vi "run_experiment_sCMOS_DAC_DEBUG.vi"() -> ()   [LabVIEW 2015]
uses:
  <vilib>/DAQmx/read.llb/DAQmx Read (Analog 1D Wfm NChan NSamp).vi
  <vilib>/DAQmx/write.llb/DAQmx Write (Digital Bool 1Line 1Point).vi
  <vilib>/DAQmx/create/channels.llb/DAQmx Create Channel (DO-Digital Output).vi
  <vilib>/DAQmx/miscellaneous.llb/DAQmx Fill In Error Info.vi
  <vilib>/DAQmx/create/channels.llb/DAQmx Create Channel (AI-Voltage-Basic).vi
  <vilib>/DAQmx/configure/timing.llb/DAQmx Timing (Sample Clock).vi
panel:
  out "Display":T1(plugin-control)
  out "DAC Input":waveform(dbl)[](graph) caption="DAC Input Display"
  out "Frames Recorded":i32
  out "error out":errorcluster
  out "Current Stimulus Name":string
  out "Current Piezo Command":dynamicdata(graph)
  out "Acquiring Frames":bool
  out "Current Stim Frames":dbl
  out "Current Stim Duration":dbl
  out "Current Stimulus Save Path":path
  in  "Number Reps":dbl
  out "Experiment Path":path
  out "Timestamp":string
  out "Genotype":string
  out "Fly Name":string
  out "Experiment Name":string
  in  "Metadata Path":path
  out "Stimulus Files":path[](array[path])
  out "Num Stimuli":i32
  out "Protocol Name":string
  out "Protocol Rate":i32
  in  "Protocol Path":path
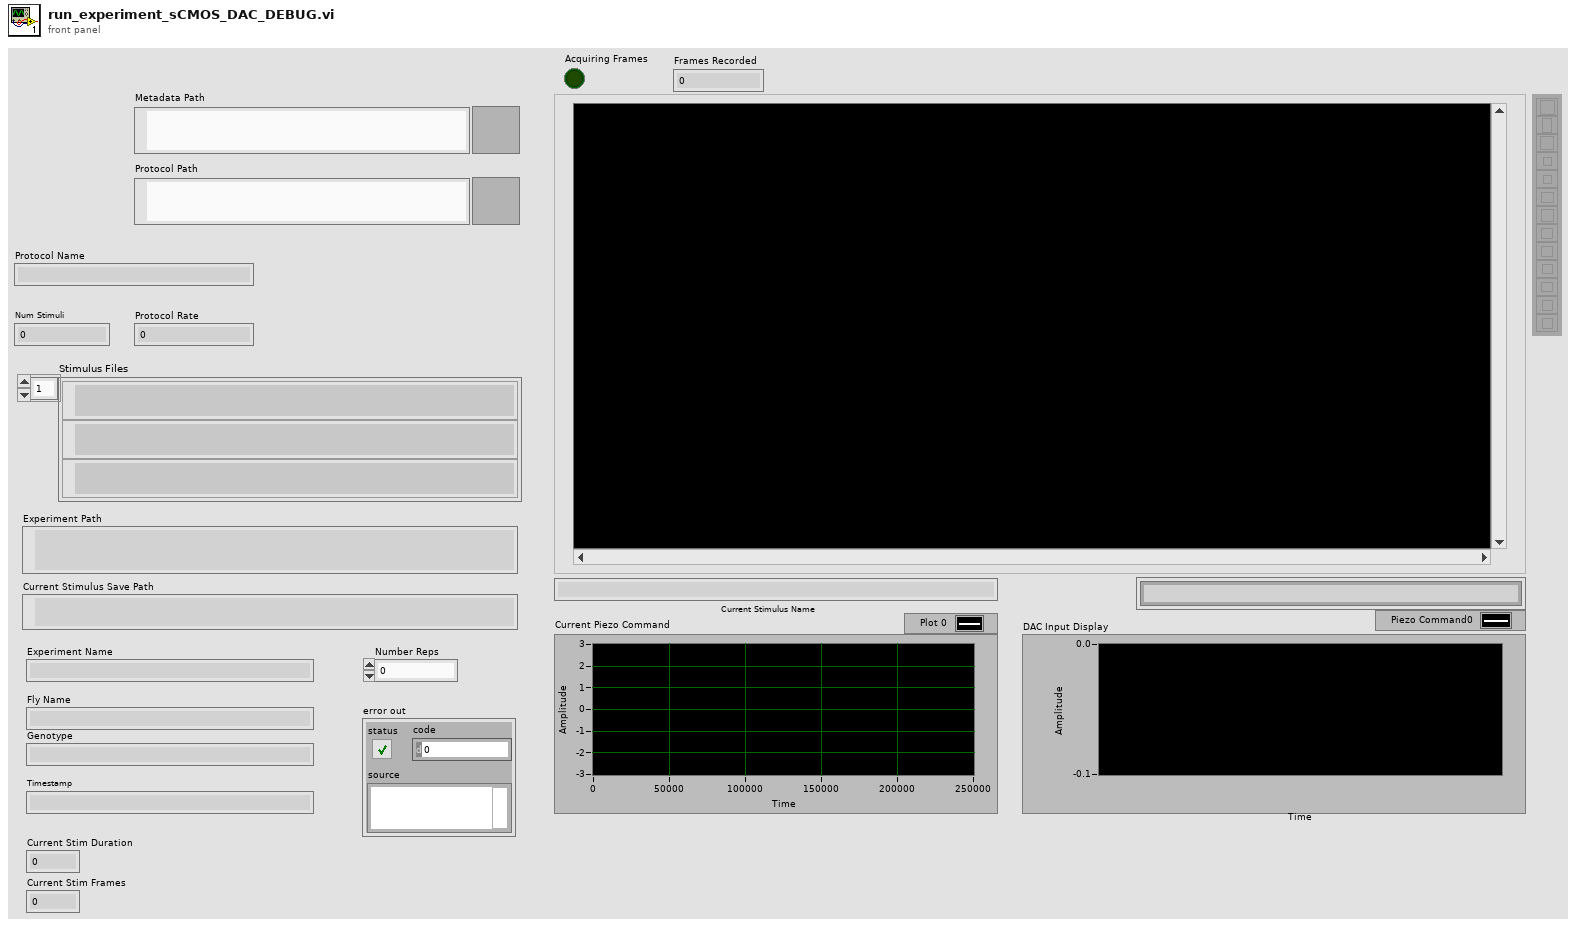
[diagram p1: front panel]
types:
  T1 = typedef "IMAQ Image.ctl" = refnum<image>
  T2 = cluster{"Value":i32, "Minimum":i32, "Maximum":i32, "Increment":i32}
  T3 = typedef "Image Type" = u32
  T4 = cluster{"height":u32, "width":u32, "datatype":u32}
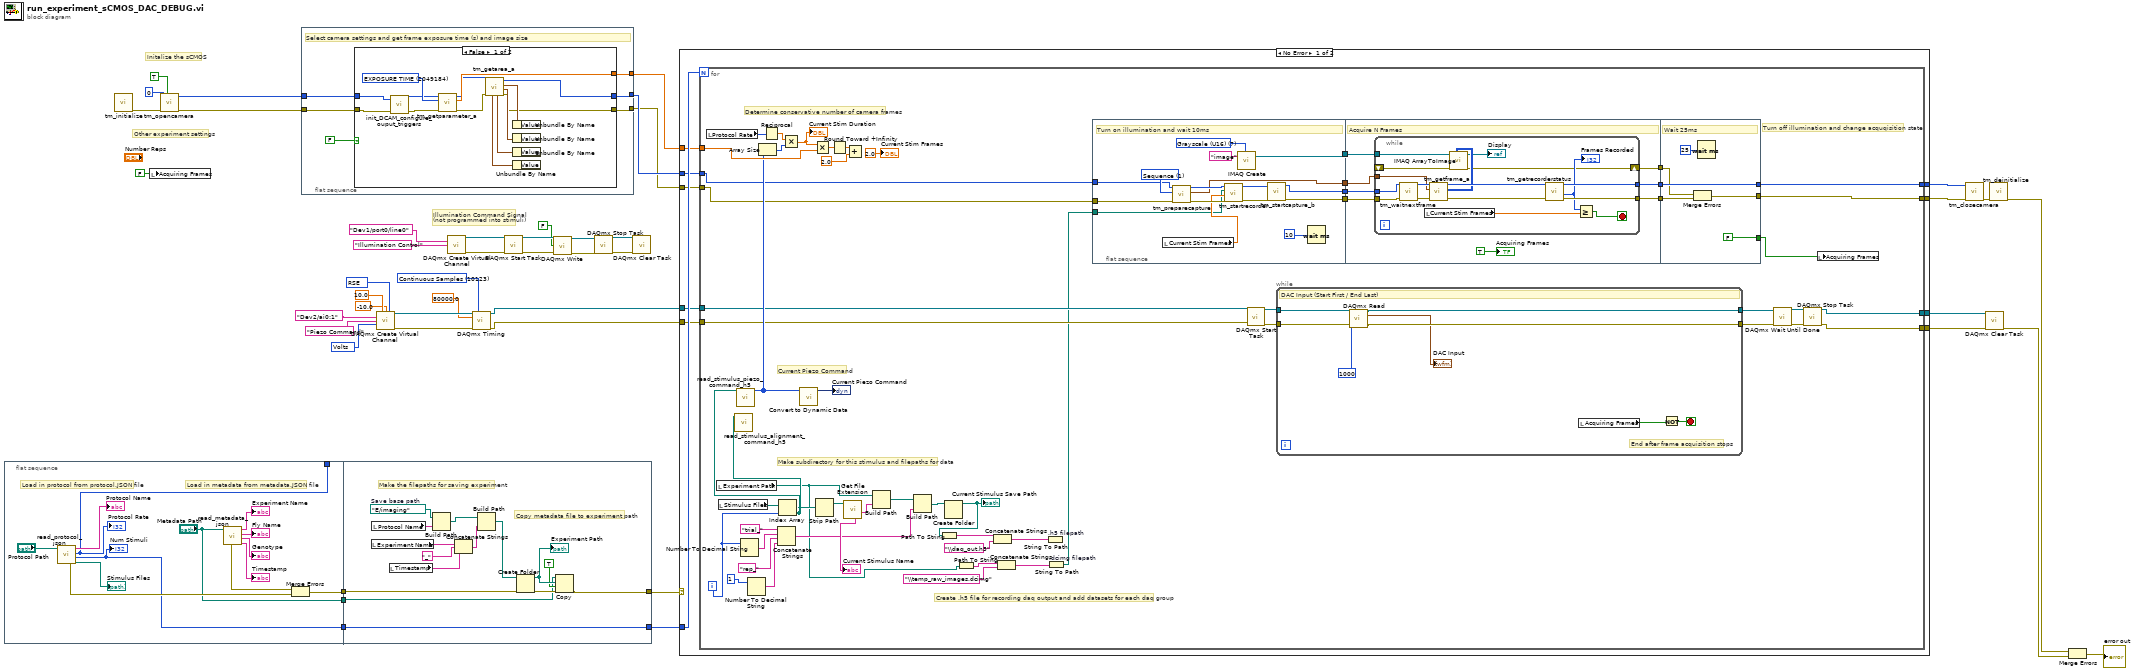
[diagram p0: block diagram]
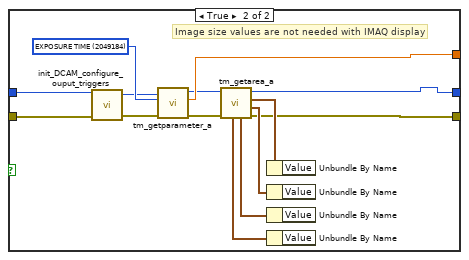
[diagram p3: hidden frame]
diagram:
  w8 = 10083 items=["default"=-1, "RSE"=10083, "NRSE"=10078, "Differential"=10106, "Pseudodifferential"=12529] ("input terminal configuration")
  w9 = 10123 items=["Finite Samples"=10178, "Continuous Samples"=10123] ("sample mode")
  w10 = 10348 items=["Volts"=10348, "From Custom Scale"=10065] ("units")
  # "Other experiment settings"
  # "Initalize the sCMOS"
  # "Illumination Command Signal \n(not programmed into stimuli)"
  n1 = flat-sequence {
    tunnel: [w48] -> _
    tunnel: [w49] -> w21
    tunnel: ["Metadata Path"] -> w20
    tunnel: [w46] -> w19
    tunnel: [w73] -> w39
    tunnel: w21 -> [w61]
    tunnel: w20 -> [w60]
    tunnel: w19 -> [w73]
    tunnel: [w59] -> w18
    frame #0 {
      # "Load in metadata from metadata.JSON file"
      # "Load in protocol from protocol.JSON file"
      n2 = call "read_protocol_json.vi"("Path"="Protocol Path") -> ("stims"=→"Stimulus Files":path[], "n_stims"=w46:i32, "rate"=w48:i32, "protocol name"=→"Protocol Name":string, "error out"=w51:errorcluster)  [unwired: 6 in]
      "Protocol Rate" <- w48
      "Num Stimuli" <- w46
      n3 = call "read_metadata_json.vi"("Path"="Metadata Path") -> ("exp_time"=→"Timestamp":string, "genotype"=→"Genotype":string, "fly_name"=→"Fly Name":string, "exp_ name"=→"Experiment Name":string, "error out"=w50:errorcluster)  [unwired: 6 in]
      n4 = Merge Errors(w50, w51) -> (w49:errorcluster)
    }
    frame #1 {
      w68 = path "E:/imaging"  # Save base path
      # "Copy metadata file to experiment path"
      # "Make the filepaths for saving experiment"
      n5 = local read "Experiment Name"() -> (w65:string)
      n6 = local read "Protocol Name"() -> (w67:string)
      n7 = local read "Timestamp"() -> (w63:string)
      n8 = Build Path(base path=w68, name or relative path=w67) -> (appended path=w66:path)
      n9 = Concatenate Strings(w65, "_", w63) -> (w62:string)
      n10 = Build Path(base path=w66, name or relative path=w62) -> (appended path=w69:path)
      n11 = Create Folder(path (use dialog)=w69, error in=w61) -> (created path=w72:path, error out=w71:errorcluster)  [unwired: 1 in, 1 out]
      "Experiment Path" <- w72
      n12 = Copy(8:w71, 9:TRUE ("overwrite (F)"), 10:w72, 11:w60) -> (0:w59:errorcluster)  [unwired: 1 in, 2 out]
    }
  }
  n13 = call <userlib>:"tm_initialize.vi"() -> ("error out"=w42:errorcluster)  [unwired: 8 in, 3 out]
  n14 = local write "Acquiring Frames"(FALSE ("Acquiring Frames")) -> ()
  n15 = call <userlib>:"tm_opencamera.vi"("Force Open"=TRUE, "error in (no error)"=w42, "Camera Index"=0) -> ("error out"=w29:errorcluster, "Handle out"=w30:u32)  [unwired: 6 in, 1 out]
  n16 = flat-sequence {
    tunnel: [w76] -> w32
    tunnel: [w75] -> w24
    tunnel: [w79] -> w31
    tunnel: w30 -> [w78]
    tunnel: w29 -> [w77]
    frame #0 {
      # "Select camera settings and get frame exposure time (s) and image size"
      n17 = case shown="False" FALSE {
        tunnel: [w92 w106] -> w79
        tunnel: w78 -> [w80 w97]
        tunnel: w77 -> [w83 w96]
        tunnel: [w85 w95] -> w76
        tunnel: [w84 w94] -> w75
        frame False {
          w93 = u32 2049184 items=["SENSOR MODE"=4212128, "CCD MODE"=4212384, "READOUT MODE"=4211872, "ACTIVE VIEW INDEX"=4343136, "BITS PER CHANNEL"=4342976, "IMAGE PIXEL TYPE"=4343296, "BINNING"=4215968, "EXPOSURE TIME"=2049184, "CONTRAST GAIN"=3163312, "CONTRAST OFFSET"=3163328, "LIGHT MODE"=2114720, "SENSITIVITY"=2114992, "PHOTON IMAGING MODE"=2115200, "HIGH DYNAMIC RANGE MODE"=3163360, "WHITE BALANCE"=3163568, "TEMPERATURE"=2115232, "TEMPERATURE TARGET"=2115264, "SENSOR COOLER FAN"=2115296, "LINEBUNDLE HEIGHT"=4212192, "MECHANICAL SHUTTER"=2115488, "BACK FOCUS POSITION"=8422304, "TRIGGER CONNECTOR"=1066432, "TRIGGER SOURCE"=1066144, "OUTPUT TRIGGER SOURCE"=1852576, "TRIGGER GLOBAL EXPOSURE"=2049680, "FIRST TRIGGER BEHAVIOR"=2049696, "CHANNEL SYNC"=1852352, "READOUT DIRECTION"=4211904, "PRE HSYNC COUNT"=1852704] ("Parameter")
          n18 = call "init_DCAM_configure_ouput_triggers.vi"("error in (no error)"=w83, "Handle in"=w80) -> ("error out"=w82:errorcluster, "Handle out"=w81:u32)  [unwired: 2 in]
          n19 = call <userlib>:"tm_getparameter_a.vi"("error in (no error)"=w82, "Parameter"=w93, "Handle in"=w81) -> ("error out"=w87:errorcluster, "Value out"=w92:dbl, "Handle out"=w86:u32)  [unwired: 6 in]
          n20 = call <userlib>:"tm_getarea_a.vi"("error in (no error)"=w87, "Handle in"=w86) -> ("error out"=w84:errorcluster, "V Offset"=w90:T2, "H Offset"=w91:T2, "Handle out"=w85:u32, "H Width"=w89:T2, "V Width"=w88:T2)  [unwired: 4 in]
          n21 = Unbundle By Name(w91) -> ()  [unwired: 1 out]
          n22 = Unbundle By Name(w90) -> ()  [unwired: 1 out]
          n23 = Unbundle By Name(w89) -> ()  [unwired: 1 out]
          n24 = Unbundle By Name(w88) -> ()  [unwired: 1 out]
        }
        frame True {
          w107 = u32 2049184 items=["SENSOR MODE"=4212128, "CCD MODE"=4212384, "READOUT MODE"=4211872, "ACTIVE VIEW INDEX"=4343136, "BITS PER CHANNEL"=4342976, "IMAGE PIXEL TYPE"=4343296, "BINNING"=4215968, "EXPOSURE TIME"=2049184, "CONTRAST GAIN"=3163312, "CONTRAST OFFSET"=3163328, "LIGHT MODE"=2114720, "SENSITIVITY"=2114992, "PHOTON IMAGING MODE"=2115200, "HIGH DYNAMIC RANGE MODE"=3163360, "WHITE BALANCE"=3163568, "TEMPERATURE"=2115232, "TEMPERATURE TARGET"=2115264, "SENSOR COOLER FAN"=2115296, "LINEBUNDLE HEIGHT"=4212192, "MECHANICAL SHUTTER"=2115488, "BACK FOCUS POSITION"=8422304, "TRIGGER CONNECTOR"=1066432, "TRIGGER SOURCE"=1066144, "OUTPUT TRIGGER SOURCE"=1852576, "TRIGGER GLOBAL EXPOSURE"=2049680, "FIRST TRIGGER BEHAVIOR"=2049696, "CHANNEL SYNC"=1852352, "READOUT DIRECTION"=4211904, "PRE HSYNC COUNT"=1852704] ("Parameter")
          # "Image size values are not needed with IMAQ display"
          n25 = call "init_DCAM_configure_ouput_triggers.vi"("error in (no error)"=w96, "Handle in"=w97) -> ("error out"=w105:errorcluster, "Handle out"=w104:u32)  [unwired: 2 in]
          n26 = call <userlib>:"tm_getparameter_a.vi"("error in (no error)"=w105, "Parameter"=w107, "Handle in"=w104) -> ("error out"=w102:errorcluster, "Value out"=w106:dbl, "Handle out"=w103:u32)  [unwired: 6 in]
          n27 = call <userlib>:"tm_getarea_a.vi"("error in (no error)"=w102, "Handle in"=w103) -> ("error out"=w94:errorcluster, "V Offset"=w100:T2, "H Offset"=w101:T2, "Handle out"=w95:u32, "H Width"=w99:T2, "V Width"=w98:T2)  [unwired: 4 in]
          n28 = Unbundle By Name(w101) -> ()  [unwired: 1 out]
          n29 = Unbundle By Name(w100) -> ()  [unwired: 1 out]
          n30 = Unbundle By Name(w99) -> ()  [unwired: 1 out]
          n31 = Unbundle By Name(w98) -> ()  [unwired: 1 out]
        }
      }
    }
  }
  n32 = call-poly <vilib>:"DAQmx Create Virtual Channel.vi"("maximum value"=10.0, "minimum value"=-10.0, "input terminal configuration"=w8, "physical channels"=tag "Dev2/ai0:1" ("DAQmx Physical Channel"), "name to assign"="Piezo Command", "units"=w10) -> ("task out"=w16:refnum<k21>, "error out"=w17:errorcluster)  [unwired: 8 in]
  n33 = call-poly <vilib>:"DAQmx Create Virtual Channel.vi"("lines"=tag "Dev1/port0/line0" ("DAQmx Physical Channel"), "name to assign"="Illumination Control") -> ("task out"=w36:refnum<k21>, "error out"=w38:errorcluster)  [unwired: 12 in]
  n34 = call-poly <vilib>:"DAQmx Timing.vi"("task/channels in"=w16, "sample mode"=w9, "rate"=80000.0, "error in"=w17) -> ("task out"=w7:refnum<k21>, "error out"=w6:errorcluster)  [unwired: 10 in]
  n35 = call <vilib>:"DAQmx Start Task.vi"("task/channels in"=w36, "error in"=w38) -> ("task out"=w35:refnum<k21>, "error out"=w37:errorcluster)  [unwired: 12 in]
  n36 = call-poly <vilib>:"DAQmx Write.vi"("task/channels in"=w35, "data"=FALSE, "error in"=w37) -> ("task out"=w5:refnum<k21>, "error out"=w4:errorcluster)  [unwired: 10 in, 1 out]
  n37 = call <vilib>:"DAQmx Stop Task.vi"("task/channels in"=w5, "error in"=w4) -> ("task out"=w2:refnum<k21>, "error out"=w3:errorcluster)  [unwired: 12 in]
  n38 = call <vilib>:"DAQmx Clear Task.vi"("task in"=w2, "error in"=w3) -> ()  [unwired: 13 in, 1 out]
  n39 = case shown="No Error" w18 {
    tunnel: w39 -> [w117 _]
    tunnel: w31 -> [w116 _]
    tunnel: w32 -> [w115 w230]
    tunnel: w24 -> [w114 w229]
    tunnel: [w113 w229] -> w26
    tunnel: [w112 w230] -> w25
    tunnel: [w111 _] -> w23
    tunnel: [w110 _] -> w22
    tunnel: w7 -> [w109 _]
    tunnel: w6 -> [w108 _]
    frame No Error {
      n40 = for {
        N: w117 -> [_]
        tunnel: w116 -> [w161]
        tunnel: w115 -> [w131]
        tunnel: w114 -> [w130]
        tunnel: [w147] -> w113
        tunnel: [w146] -> w112
        tunnel: [w136] -> w111
        tunnel: [w135] -> w110
        tunnel: w109 -> [w134]
        tunnel: w108 -> [w133]
        i -> [w170]
        # "Create .h5 file for recording daq output and add datasets for each daq group"
        # "Current Piezo Command"
        # "Turn off illumination and change acquqisition state"
        # "Determine conservative number of camera frames"
        # "Make subdirectory for this stimulus and filepaths for data"
        n41 = local read "Protocol Rate"() -> (w165:i32)
        n42 = local read "Experiment Path"() -> (w122:path)
        n43 = local read "Stimulus Files"() -> (w171:path[])
        n44 = Number To Decimal String(number=w170) -> (decimal integer string=w173:string)  [unwired: 1 in]
        n45 = Number To Decimal String(number=i16 1 ("width (-)")) -> (decimal integer string=w168:string)  [unwired: 1 in]
        n46 = Reciprocal(x=w165) -> (1/x=w163:dbl)
        n47 = Concatenate Strings("trial_", w173, "rep_", w168) -> (w123:string)
        n48 = Index Array(array=w171, index=w170) -> (element=w166:path)
        n49 = call "read_stimulus_alignment_command_h5.vi"("Path"=w166) -> ()  [unwired: 9 in, 2 out]
        n50 = call "read_stimulus_piezo_command_h5.vi"("Path"=w166) -> ("stimulus"=w141:i32[])  [unwired: 9 in, 1 out]
        n51 = Array Size(array=w141) -> (size(s)=w164:i32)
        n52 = Multiply(x=w163, y=w164) -> (x*y=w162:dbl)
        "Current Stim Duration" <- w162
        n53 = call "Convert to Dynamic Data"("Array"=w141) -> ("Dynamic Data Type"=→"Current Piezo Command":dynamicdata)  [unwired: 3 in]
        n54 = Multiply(x=w162, y=w161) -> (x*y=w160:dbl)
        n55 = Strip Path(path=w166) -> (stripped path=w129:path)  [unwired: 1 out]
        n56 = Round Toward +Infinity(x=w160) -> (ceil(x): smallest int >= x=w159:dbl)
        n57 = call <vilib>:"Get File Extension.vi"("file"=w129) -> ("filename without extension"=w128:string, "unmodified file extension"=→"Current Stimulus Name":string)  [unwired: 6 in, 3 out]
        n58 = Add(x=w159, y=2.0) -> ()  [unwired: 1 out]
        n59 = Build Path(base path=w122, name or relative path=w128) -> (appended path=w125:path)
        n60 = Build Path(base path=w125, name or relative path=w123) -> (appended path=w124:path)
        n61 = Create Folder(path (use dialog)=w124) -> (created path=w126:path)  [unwired: 2 in, 2 out]
        "Current Stimulus Save Path" <- w126
        n62 = Path To String(path=w126) -> (string=w156:string)
        n63 = Path To String(path=w122) -> (string=w121:string)
        n64 = Concatenate Strings(w156, "\\daq_out.h5" ("string")) -> (w157:string)
        n65 = Concatenate Strings(w121, "\\temp_raw_images.dcimg" ("string")) -> (w119:string)
        n66 = String To Path ".h5 filepath"(string=w157) -> ()  [unwired: 1 out]
        n67 = String To Path ".dcimg filepath"(string=w119) -> (path=w118:path)
        n68 = flat-sequence {
          tunnel: [w181] -> w152
          tunnel: [w179] -> w151
          tunnel: [w180] -> w150
          tunnel: [w175] -> w143
          tunnel: w131 -> [w187]
          tunnel: w130 -> [w186]
          tunnel: w118 -> [w174]
          tunnel: w152 -> [w196]
          tunnel: w151 -> [w195]
          tunnel: w150 -> [w194]
          tunnel: [w193] -> w149
          tunnel: [w192] -> w148
          tunnel: w143 -> [w191]
          tunnel: [w190] -> w142
          tunnel: [FALSE] -> w154
          tunnel: w149 -> [w218]
          tunnel: w148 -> [w216]
          tunnel: [w217] -> w147
          tunnel: [w218] -> w146
          tunnel: w142 -> [w215]
          frame #0 {
            w177 = T3 7 items=["Grayscale (U8)", "Grayscale (I16)", "Grayscale (SGL)", "Complex (CSG)", "RGB (U32)", "HSL (U32)", "RGB (U64)", "Grayscale (U16)"] ("Image Type")
            w188 = 1 items=["Snap", "Sequence"] ("Capture mode")
            # "Turn on illumination and wait 10ms"
            n69 = local read "Current Stim Frames"() -> (w178:dbl)
            n70 = call <userlib>:"tm_preparecapture.vi"("error in (no error)"=w186, "Capture mode"=w188, "Handle in"=w187) -> ("error out"=w185:errorcluster, "Buffer Info"=w179:T4, "Handle out"=w184:u32)  [unwired: 5 in, 1 out]
            n71 = call <userlib>:"tm_startrecorder.vi"("error in (no error)"=w185, "frames"=w178, "File"=w174, "Handle in"=w184) -> ("error out"=w182:errorcluster, "Handle out"=w183:u32)  [unwired: 6 in]
            n72 = call "IMAQ Create"("Image Name"="image", "Image Type"=w177) -> ("New Image"=w175:T1)  [unwired: 3 in, 1 out]
            n73 = call <userlib>:"tm_startcapture_b.vi"("error in (no error)"=w182, "Handle in"=w183) -> ("error out"=w181:errorcluster, "Handle out"=w180:u32)  [unwired: 8 in]
            n74 = Wait (ms)(milliseconds to wait=u32 10) -> ()  [unwired: 1 out]
          }
          frame #1 {
            # "Acquire N Frames"
            n75 = while {
              tunnel: w196 -> [w210]
              tunnel: w195 -> [w209]
              tunnel: w194 -> [w208]
              tunnel: [w207] -> w193
              tunnel: [w206] -> w192
              tunnel: w191 -> [w202]
              shift-right: [w200] -> w190
              shift-left: _ -> [w199]
              stop <- w203 stop-if-true
              n76 = call <userlib>:"tm_waitnextframe.vi"("error in (no error)"=w210, "Handle in"=w208) -> ("error out"=w212:errorcluster, "Handle out"=w211:u32)  [unwired: 6 in, 2 out]
              n77 = local read "Current Stim Frames"() -> (w204:dbl)
              n78 = call <userlib>:"tm_getframe_a.vi"("error in (no error)"=w212, "Buffer Info"=w209, "Handle in"=w211) -> ("error out"=w213:errorcluster, "Data 16"=w201:u16[][], "Handle out"=w214:u32)  [unwired: 4 in, 2 out]
              n79 = call "IMAQ ArrayToImage"("Image Pixels (U16)"=w201, "error in (no error)"=w199, "Image"=w202) -> ("error out"=w200:errorcluster, "Image Out"=→"Display":T1)  [unwired: 7 in]
              n80 = call <userlib>:"tm_getrecorderstatus.vi"("error in (no error)"=w213, "Handle"=w214) -> ("error out"=w206:errorcluster, "Count"=w205:i32, "Handle"=w207:u32)  [unwired: 6 in, 1 out]
              "Frames Recorded" <- w205
              n81 = Greater Or Equal?(x=w205, y=w204) -> (x >= y?=w203:bool)
            }
            "Acquiring Frames" <- TRUE
          }
          frame #2 {
            # "Wait 25ms"
            n82 = Merge Errors(w215, w216) -> (w217:errorcluster)
            n83 = Wait (ms)(milliseconds to wait=u32 25) -> ()  [unwired: 1 out]
          }
        }
        n84 = call <vilib>:"DAQmx Start Task.vi"("task/channels in"=w134, "error in"=w133) -> ("task out"=w145:refnum<k21>, "error out"=w144:errorcluster)  [unwired: 12 in]
        n85 = while {
          tunnel: w144 -> [w224]
          tunnel: [w227] -> w137
          tunnel: w145 -> [w225]
          tunnel: [w226] -> w138
          stop <- w228 stop-if-true
          # "End after frame acquisition stops"
          # "DAC Input (Start First / End Last)"
          n86 = call-poly <vilib>:"DAQmx Read.vi"("task/channels in"=w225, "number of samples per channel"=1000, "error in"=w224) -> ("task out"=w226:refnum<k21>, "data"=→"DAC Input":waveform(dbl)[], "error out"=w227:errorcluster)  [unwired: 10 in]
          n87 = local read "Acquiring Frames"() -> (w222:bool)
          n88 = Not(x=w222) -> (.not. x?=w228:bool)
        }
        n89 = call <vilib>:"DAQmx Wait Until Done.vi"("task/channels in"=w138, "error in"=w137) -> ("task out"=w140:refnum<k21>, "error out"=w139:errorcluster)  [unwired: 12 in]
        n90 = call <vilib>:"DAQmx Stop Task.vi"("task/channels in"=w140, "error in"=w139) -> ("task out"=w135:refnum<k21>, "error out"=w136:errorcluster)  [unwired: 12 in]
        n91 = local write "Acquiring Frames"(w154) -> ()
        "Current Stim Frames" <- 2.0 ("Current Stim Frames")
      }
    }
    frame Error {
    }
  }
  n92 = call <userlib>:"tm_closecamera.vi"("error in (no error)"=w26, "Handle in"=w25) -> ("error out"=w28:errorcluster)  [unwired: 9 in]
  n93 = call <vilib>:"DAQmx Clear Task.vi"("task in"=w22, "error in"=w23) -> ("error out"=w1:errorcluster)  [unwired: 13 in]
  n94 = call <userlib>:"tm_deinitialize.vi"("error in (no error)"=w28) -> ("error out"=w27:errorcluster)  [unwired: 10 in]
  n95 = Merge Errors(w27, w1) -> (→"error out":errorcluster)
